vi "Stop.vi"(8 "error in (no error)":errorcluster, 11 "Virt Instr Base in":refnum<class "Virt Instr Host.lvclass">) -> (0 "error out":errorcluster, 3 "Virt Instr Base out":refnum<class "Virt Instr Host.lvclass">)   [LabVIEW 2023, in "HAL GOOP4.lvlib" / "Virt Instr Host.lvclass"]
uses:
  Virt Instr Host.lvclass
  Virt Instr Host.lvclass/Virt Instr Host.ctl
  Instrument/Instrument.lvclass
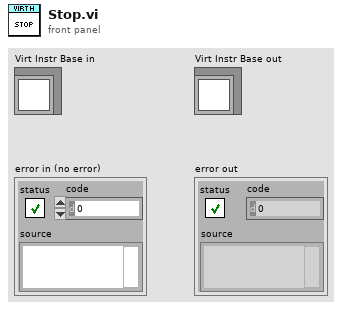
[diagram p1: front panel]
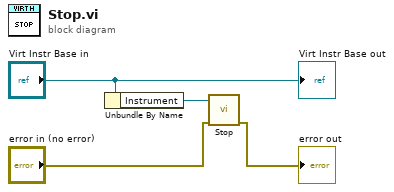
[diagram p0: block diagram]
diagram:
  n1 = Unbundle By Name("Virt Instr Base in") -> ("Instrument"=w3:refnum<class "Instrument.lvclass">)
  n2 = call "Stop.vi"("error in (no error)"="error in (no error)", "reference in"=w3) -> ("error out"=→"error out":errorcluster)  [unwired: 8 in, 1 out]
  "Virt Instr Base out" <- "Virt Instr Base in"
